vi "Log Status Update.vi"(8 "error in (no error)":errorcluster, 10 "String":string, 11 "TestStand Controller in":refnum<class "Controller API.lvclass">) -> (0 "error out":errorcluster, 3 "TestStand Controller out":refnum<class "Controller API.lvclass">)   [LabVIEW 2016, in "Controller API.lvlib" / "Controller API.lvclass"]
uses:
  Controller API.lvclass
  Controller API.lvclass/Controller API.ctl
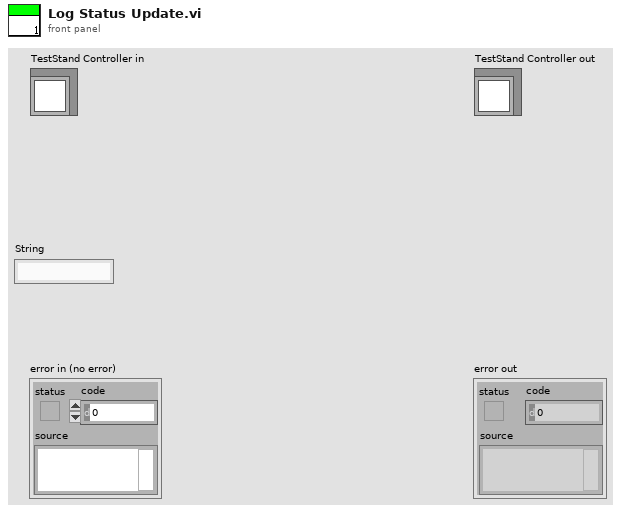
[diagram p1: front panel]
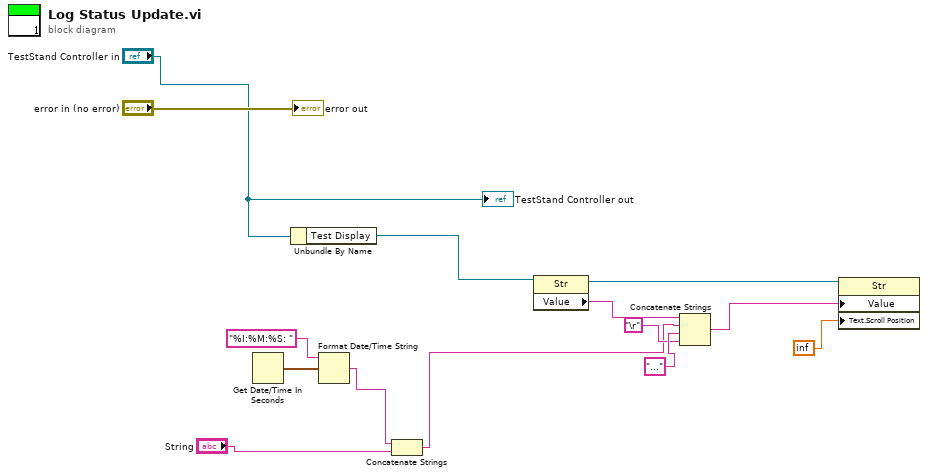
[diagram p0: block diagram]
diagram:
  n1 = Get Date/Time In Seconds() -> (seconds since 1Jan1904=w6:timestamp)
  n2 = Unbundle By Name("TestStand Controller in") -> ("Test Display"=w2:refnum<vi>)
  n3 = Format Date/Time String(time format string (%c)="%I:%M:%S: ", seconds (now)=w6) -> (date/time string=w4:string)  [unwired: 1 in]
  n4 = Concatenate Strings(w4, "String") -> (w7:string)
  n5 = property class="Str"(reference=w2) -> (reference out=w13:refnum<vi>, "Value"=w12:string)  [unwired: 1 in, 1 out]
  n6 = Concatenate Strings(w12, w7, "..." ("string"), "\r") -> (w11:string)
  n7 = property class="Str"(reference=w13, "Value"=w11, "Text.Scroll Position"=inf) -> ()  [unwired: 1 in, 2 out]
  "error out" <- "error in (no error)"
  "TestStand Controller out" <- "TestStand Controller in"
